vi "Array of Variants to Variant Cluster.vi"(8 "error in (no error)":errorcluster, 11 "Array":variant[](array[variant])) -> (0 "error out":errorcluster, 3 "VCluster":variant)   [LabVIEW 2017, in "JSON Value.lvclass"]
uses:
  JSON Value.lvclass
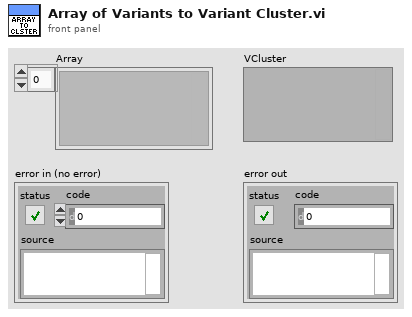
[diagram p1: front panel]
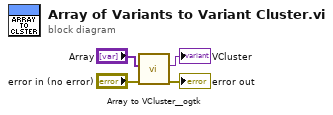
[diagram p0: block diagram]
diagram:
  n1 = call "Array to VCluster__ogtk.vi"("error in (no error)"="error in (no error)", "Array"="Array") -> ("error out"=→"error out":errorcluster, "VCluster"=→"VCluster":variant)  [unwired: 8 in]
